vi "ArcadeDriveCurve.vi"(9 "Direction":dbl format="%#_13g", 10 "Throttle":dbl format="%#_13g", 11 "Deadzone":dbl format="%#_13g") -> (1 "DriveRight":dbl, 2 "DriveLeft":dbl)   [LabVIEW 2015]
doc: "Based on the given throttle and direction, sets the left and right motor outputs. If direction is within deadzone, both motor outputs are zero. If direction is outside deadzone, the throttle is assigned to one side (depending on the sign of direction), while the other side is scaled according to a cosine function: scale = cos(pi*abs(direction))."
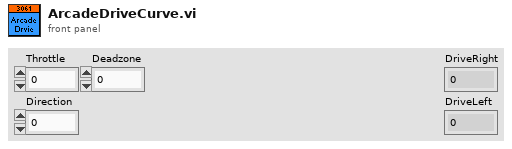
[diagram p1: front panel]
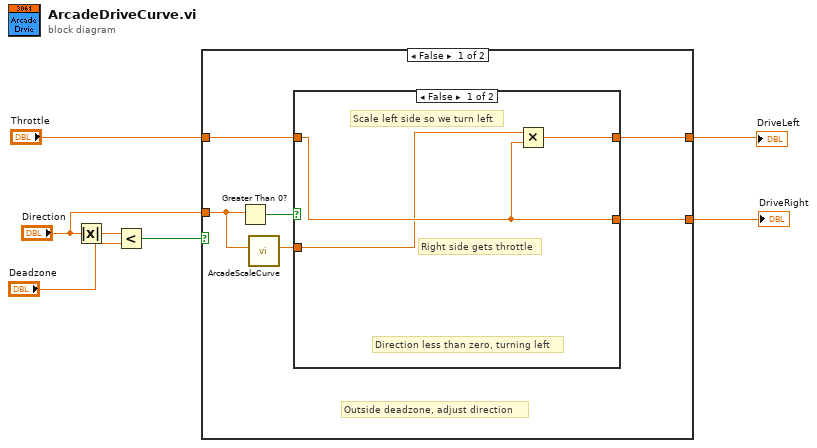
[diagram p0: block diagram]
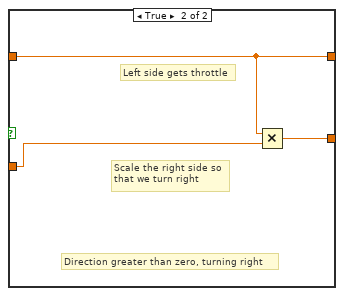
[diagram p2: hidden frame]
diagram:
  n1 = Absolute Value(x="Direction") -> (abs(x)=w6:dbl)
  n2 = Less?(x=w6, y="Deadzone") -> (x < y?=w4:bool)
  n3 = case shown="False" w4 {
    tunnel: "Throttle" -> [w13 w20]
    tunnel: [w11 w20] -> w2
    tunnel: [w8 w20] -> w3
    tunnel: "Direction" -> [w10 _]
    frame False {
      # "Outside deadzone, adjust direction"
      n4 = Greater Than 0?(x=w10) -> (x > 0?=w12:bool)
      n5 = call "ArcadeScaleCurve.vi"("Direction"=w10) -> ("Scale"=w9:dbl)  [unwired: 10 in]
      n6 = case shown="False" w12 {
        tunnel: w13 -> [w16 w19]
        tunnel: [w14 w19] -> w11
        tunnel: w9 -> [w15 w18]
        tunnel: [w16 w17] -> w8
        frame False {
          # "Scale left side so we turn left"
          # "Right side gets throttle"
          # "Direction less than zero, turning left"
          n7 = Multiply(x=w15, y=w16) -> (x*y=w14:dbl)
        }
        frame True {
          # "Scale the right side so\nthat we turn right"
          # "Left side gets throttle"
          # "Direction greater than zero, turning right"
          n8 = Multiply(x=w19, y=w18) -> (x*y=w17:dbl)
        }
      }
    }
    frame True {
      # "Within deadzone, act like straight drive"
    }
  }
  "DriveRight" <- w3
  "DriveLeft" <- w2
